vi "Run.vi"(7 "Team Index":i32, 8 "Column":i32, 9 "Row":i32, 10 "View":i32[](array[numeric]) caption="View (Team Index, -1: empty)", 11 "Atom In":refnum<class "Atom.lvclass">) -> (0 "Replicated":refnum<class "Square.lvclass">, 1 "Direction":T1, 2 "Action":T2, 3 "Square Out":refnum<class "Square.lvclass">)   [LabVIEW 2017, in "Atom.lvclass"]
uses:
  Atom.lvclass
  C:/Users/jacob/Documents/squarebattle/Square/Square.lvclass
  Square/Square.lvclass
  Type Defs/Action Enum.ctl
  Type Defs/Direction Enum.ctl
  Atom.lvclass/Atom.ctl
  SubVIs/Globals (private).vi
  SubVIs/Read-Only Stats.vi
  Type Defs/SB Type Defs.lvlib
  Common/Common.lvlib
  SubVIs/SB SubVIs.lvlib
panel:
  # "NW\nN\nNE\nE\nSE\nS\nSW\nW"
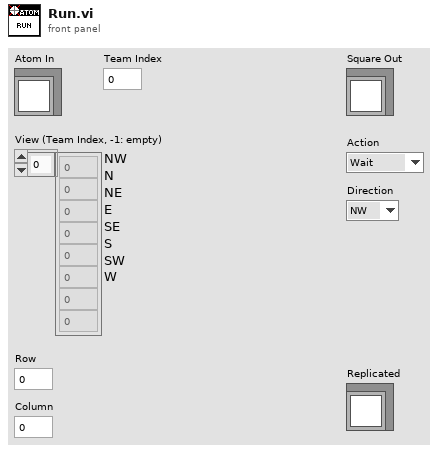
[diagram p1: front panel]
types:
  T1 = typedef "SB Type Defs.lvlib/Direction Enum.ctl" = enum16{"NW", "N", "NE", "E", "SE", "S", "SW", "W"}
  T2 = typedef "SB Type Defs.lvlib/Action Enum.ctl" = enum16{"Wait", "Move", "Attack", "Replicate"}
  T3 = typedef "Atom.lvclass/AttackMap DVR.ctl" = refnum<data-value>
  T4 = typedef "Common.lvlib/Map DVR.ctl" = refnum<data-value>
  T5 = typedef "Common.lvlib/Position.ctl" = cluster{"Column":i32, "Row":i32}
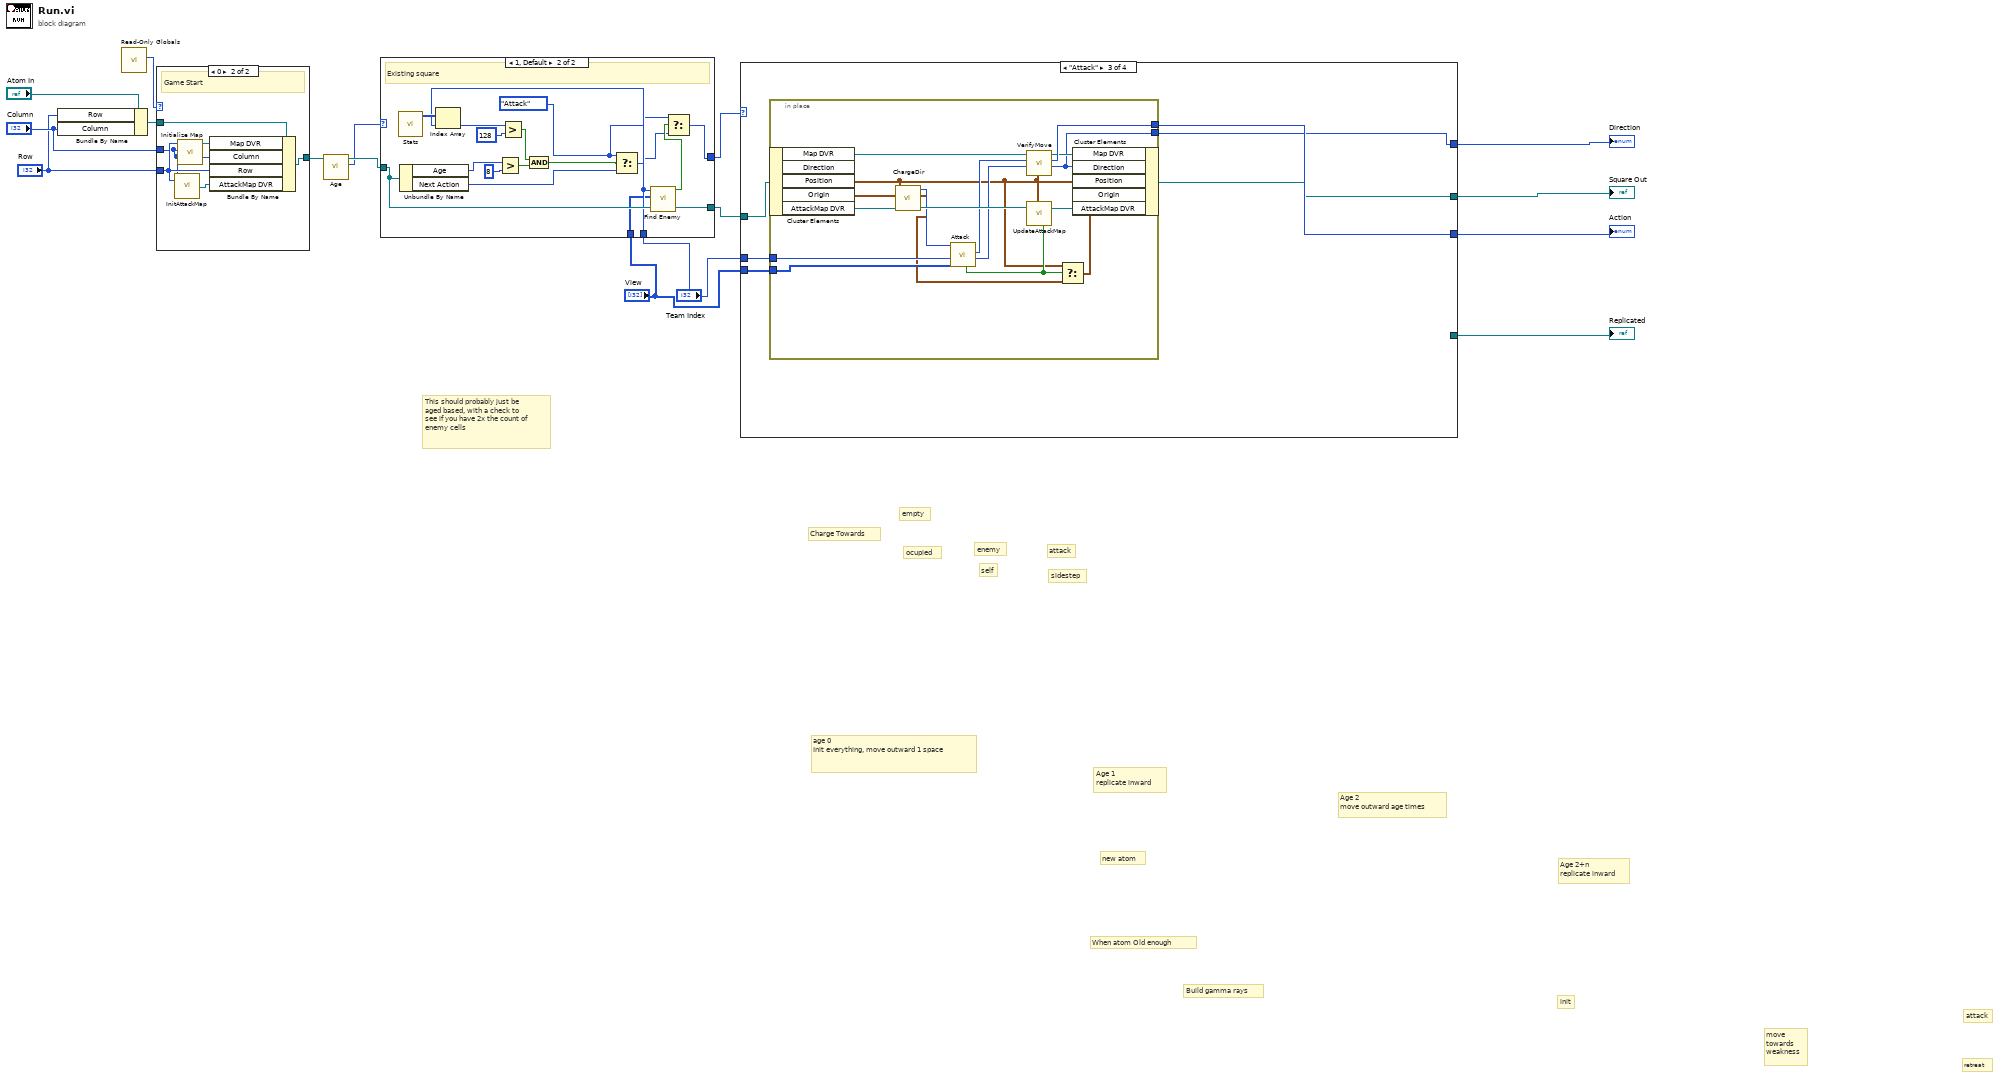
[diagram p0: block diagram]
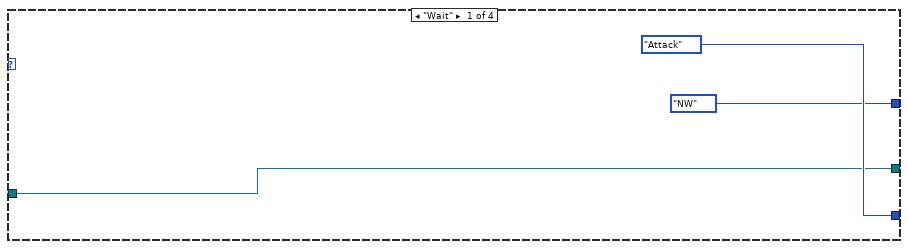
[diagram p2: hidden frame]
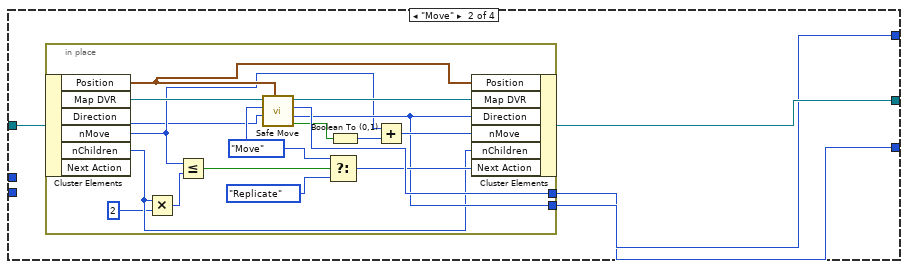
[diagram p3: hidden frame]
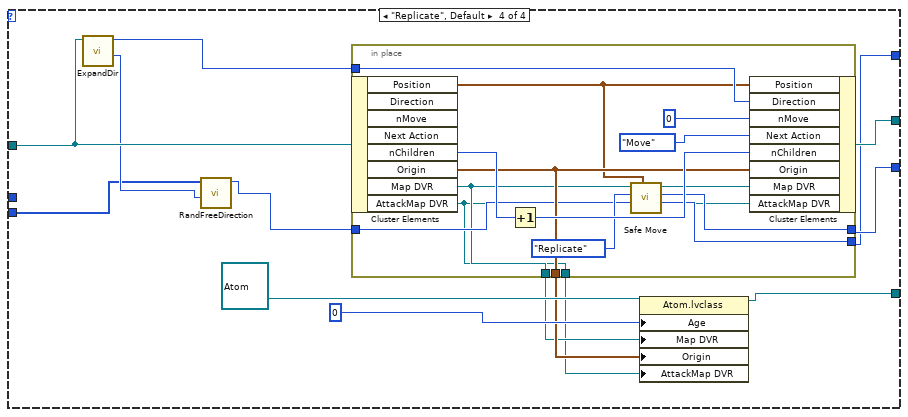
[diagram p4: hidden frame]
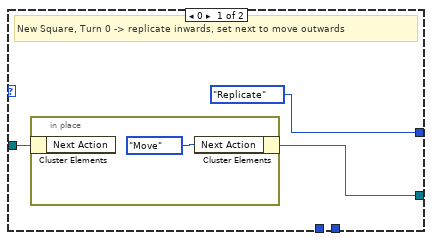
[diagram p6: hidden frame]
diagram:
  # "sidestep"
  # "attack"
  # "self"
  # "enemy"
  # "ocupied"
  # "empty"
  # "Charge Towards"
  # "This should probably just be aged based, with a check to see if you have 2x the count of enemy cells"
  # "retreat"
  # "attack"
  # "move\ntowards\nweakness"
  # "init"
  # "Build gamma rays"
  # "When atom Old enough"
  # "Age 2+n\nreplicate inward"
  # "Age 2\nmove outward age times"
  # "new atom"
  # "Age 1\nreplicate inward"
  # "age 0\nInit everything, move outward 1 space"
  n1 = Bundle By Name(cluster="Atom In", "Row"="Row", "Column"="Column") -> (w11:refnum<class "Atom.lvclass">)
  n2 = call "Read-Only Globals.vi"() -> ("Round"=w12:i32)  [unwired: 10 in, 1 out]
  n3 = case shown="0" w12 {
    tunnel: w11 -> [w17 w22]
    tunnel: [w17 w21] -> w7
    tunnel: "Row" -> [_ w19]
    tunnel: "Column" -> [_ w18]
    frame Default {
      # "Play Game"
    }
    frame 0 {
      # "Game Start"
      n4 = call "InitAttackMap.vi"("Column"=w18, "Row"=w19) -> ("AttackMap DVR"=w20:T3)
      n5 = call "Initialize Map.vi"("Column"=w18, "Row"=w19) -> ("Map DVR"=w23:T4)  [unwired: 9 in]
      n6 = Bundle By Name(cluster=w22, "Map DVR"=w23, "Column"=w18, "Row"=w19, "AttackMap DVR"=w20) -> (w21:refnum<class "Atom.lvclass">)
    }
  }
  n7 = call "Age.vi"("Atom In"=w7) -> ("Current Age"=w14:i32, "Atom Out"=w15:refnum<class "Atom.lvclass">)  [unwired: 9 in]
  n8 = case shown="1, Default" w14 {
    tunnel: [Action_Enum."Replicate" ("Next Action") w30] -> w16
    tunnel: w15 -> [w26 w43]
    tunnel: [w25 w43] -> w13
    tunnel: "Team Index" -> [_ w34]
    tunnel: "View" -> [_ w33]
    frame 0 {
      # "New Square, Turn 0 -> replicate inwards, set next to move outwards"
      n9 = in-place {
        n10 = in-place-cluster #1(w26) -> ()  [unwired: 1 out]
        n11 = in-place-cluster #1("Next Action"=Action_Enum."Move") -> (w25:refnum<class "Atom.lvclass">)
      }
    }
    frame 1, Default {
      w29 = Action_Enum."Attack" ("t")
      # "Existing square"
      n12 = call "Stats.vi"() -> ("Squares"=w40:i32[])  [unwired: 7 in, 4 out]
      n13 = Unbundle By Name(w43) -> ("Age"=w39:i32, "Next Action"=w42:T2)
      n14 = Index Array(array=w40, index=w34) -> (element=w35:i32)
      n15 = Greater?(x=w39, y=8) -> (0:w37:bool)
      n16 = Greater?(x=w35, y=128) -> (0:w36:bool)
      n17 = And(x=w36, y=w37) -> (x .and. y?=w28:bool)
      n18 = Select(t=w29, s=w28, f=w42) -> (s? t:f=w31:T2)
      n19 = call "Find Enemy.vi"("View"=w33, "Team Index"=w34) -> ("Found Enemy?"=w32:bool)  [unwired: 7 in, 2 out]
      n20 = Select(t=w29, s=w32, f=w31) -> (s? t:f=w30:T2)
    }
  }
  n21 = case shown="\"Attack\"" w16 {
    tunnel: [w45 w50 w68 w104] -> w5
    tunnel: w13 -> [w45 w49 w70 w103]
    tunnel: [Action_Enum."Attack" ("Action") w47 w72 w96] -> w3
    tunnel: [Direction_Enum."NW" ("InwardDir") w48 w71 w95] -> w6
    tunnel: "Team Index" -> [_ _ w69 _]
    tunnel: [_ _ _ w102] -> w4
    tunnel: "View" -> [_ _ w73 w91]
    frame "Wait" {
    }
    frame "Move" {
      n22 = in-place {
        in-place-border: [w67] -> w47
        in-place-border: [w58] -> w48
        w57 = Action_Enum."Move" ("Next Action")
        n23 = in-place-cluster #2(w49) -> ("Position"=w59:T5, "Map DVR"=w66:T4, "Direction"=w54:T1, "nMove"=w56:i32, "nChildren"=w53:i32)  [unwired: 1 out]
        n24 = Multiply(x=w53, y=2) -> (x*y=w52:i32)
        n25 = Less Or Equal?(x=w56, y=w52) -> (x <= y?=w64:bool)
        n26 = call "Safe Move.vi"("Position in"=w59, "Direction in"=w54, "Desired Action"=w57, "Map DVR"=w66) -> ("Accepted?"=w60:bool, "Direction"=w58:T1, "Action"=w67:T2, "Map DVR out"=w65:T4)  [unwired: 4 in]
        n27 = Select(t=w57, s=w64, f=Action_Enum."Replicate" ("Next Action")) -> (s? t:f=w62:T2)
        n28 = Boolean To (0,1)(Boolean=w60) -> (0, 1=w55:i16)
        n29 = Add(x=w56, y=w55) -> (x+y=w61:i32)
        n30 = in-place-cluster #2("Position"=w59, "Map DVR"=w65, "Direction"=w58, "nMove"=w61, "nChildren"=w53, "Next Action"=w62) -> (w50:refnum<class "Atom.lvclass">)
      }
    }
    frame "Attack" {
      n31 = in-place {
        in-place-border: w73 -> [w78]
        in-place-border: [w90] -> w72
        in-place-border: [w87] -> w71
        in-place-border: w69 -> [w79]
        n32 = in-place-cluster #3(w70) -> ("Map DVR"=w89:T4, "Position"=w76:T5, "Origin"=w86:T5, "AttackMap DVR"=w84:T3)  [unwired: 1 out]
        n33 = call "ChargeDir.vi"("AttackMap DVR In"=w84, "Origin"=w86, "Position"=w76) -> ("AttackMap DVR Out"=w83:T3, "Origin Out"=w75:T5, "Direction Of Charge"=w80:T1)  [unwired: 6 in]
        n34 = call "Attack.vi"("View"=w78, "Team Index"=w79, "ChargeDirection"=w80) -> ("Direction"=w81:i32, "Action"=w82:T2, "Enemy Found?"=w77:bool)  [unwired: 4 in, 2 out]
        n35 = call "VerifyMove.vi"("Position in"=w76, "Direction in"=w81, "Desired Action"=w82, "Map DVR"=w89) -> ("Direction"=w87:T1, "Action"=w90:T2, "Map DVR out"=w88:T4)  [unwired: 4 in, 1 out]
        n36 = call "UpdateAttackMap.vi"("Attacked?"=w77, "Position"=w76, "AttackMap DVR In"=w83) -> ("AttackMap DVR Out"=w85:T3)  [unwired: 8 in]
        n37 = Select(t=w76, s=w77, f=w75) -> (s? t:f=w74:T5)
        n38 = in-place-cluster #3("Map DVR"=w88, "Direction"=w87, "Position"=w76, "Origin"=w74, "AttackMap DVR"=w85) -> (w68:refnum<class "Atom.lvclass">)
      }
    }
    frame "Replicate", Default {
      n39 = call "ExpandDir.vi"("Atom In"=w103) -> ("InwardDir"=w92:T1, "OutwardDir"=w98:T1)  [unwired: 9 in]
      n40 = call "RandFreeDirection.vi"("Intended Dir"=w92, "View"=w91) -> ("Direction"=w94:T1)  [unwired: 8 in, 1 out]
      n41 = in-place {
        in-place-border: [w107] -> w97
        in-place-border: [w114] -> w99
        in-place-border: w98 -> [w113]
        in-place-border: w94 -> [w111]
        in-place-border: [w109] -> w96
        in-place-border: [w108] -> w95
        in-place-border: [w105] -> w93
        n42 = in-place-cluster #4(w103) -> ("Position"=w106:T5, "nChildren"=w116:i32, "Origin"=w114:T5, "Map DVR"=w107:T4, "AttackMap DVR"=w105:T3)  [unwired: 3 out]
        n43 = Increment(x=w116) -> (x+1=w115:i32)
        n44 = call "Safe Move.vi"("Position in"=w106, "Direction in"=w111, "Desired Action"=Action_Enum."Replicate" ("Action"), "Map DVR"=w107) -> ("Direction"=w108:T1, "Action"=w109:T2, "Map DVR out"=w110:T4)  [unwired: 4 in, 1 out]
        n45 = in-place-cluster #4("Position"=w106, "Direction"=w113, "nMove"=0, "Next Action"=Action_Enum."Move", "nChildren"=w115, "Origin"=w114, "Map DVR"=w110, "AttackMap DVR"=w105) -> (w104:refnum<class "Atom.lvclass">)
      }
      n46 = property class="Atom.lvclass"(reference=refnum<class "Atom.lvclass"> refnum ("Atom.lvclass"), "Age"=0, "Map DVR"=w97, "Origin"=w99, "AttackMap DVR"=w93) -> (reference out=w102:refnum<class "Atom.lvclass">)  [unwired: 1 in, 1 out]
    }
  }
  "Square Out" <- w5
  "Action" <- w3
  "Direction" <- w6
  "Replicated" <- w4
